vi "Main_v2.0.vi"() -> ()   [LabVIEW 2018]
doc: "This template is for the Queued Message Handler design pattern.\n\nThe Event Handling Loop generates messages based on user interface actions.\n\nThe Message Handling Loop processes messages generated by the Event Handling Loop, or by other messages. The messages are string values, so new messages can be added easily to the Message Cases case structure in the Message Handling Loop. Each message cluster can also provide an optional value for Message Data, which is a variant that can be converted to whatever message-specific data is required."
uses:
  Data_Type Def.ctl
  <vilib>/DAQmx/read.llb/DAQmx Read (Analog 1D DBL 1Chan NSamp).vi
  Global Variables.vi
  Enqueue Message (Single).vi
  <vilib>/measure/macond.llb/FIR Filter for 1 Chan.vi
  <vilib>/addons/Time Series Analysis/Statistical Analysis.llb/TSA Mean (Waveform).vi
  <vilib>/Utility/file.llb/Write Delimited Spreadsheet (DBL).vi
  <vilib>/DAQmx/create/channels.llb/DAQmx Create Channel (AI-Voltage-Basic).vi
  <vilib>/DAQmx/configure/timing.llb/DAQmx Timing (Sample Clock).vi
  <vilib>/DAQmx/configure/trigger.llb/DAQmx Start Trigger (Digital Edge).vi
  <vilib>/DAQmx/miscellaneous.llb/DAQmx Fill In Error Info.vi
  Message Queue.lvlib
  User Event - Stop.lvlib
  <resource>/objmgr/daqmx.rc
  <vilib>/measure/NI_MAPro.lvlib
  <vilib>/addons/_Advanced Signal Processing/NI_AdvSigProcTSA.lvlib
panel:
  out "Global Cos Corrected":T1(plugin-control)
  in  "Z dim (mm)":dbl=81.8
  out "Image array":dbl[][](array[numeric])
  in  "Experiment Name":string="v1_3x3_rep-1"
  out "Base File Name":string
  out "Points measured":i32
  in  "Trigger form CNC":tag="/DAQ2/PFI7"
  in  "Bleed (mm)":dbl=3.0
  in  "STOP":bool
  out "RAW":T1(plugin-control)
  in  "Max Input (V)":dbl=0.5
  in  "Min Input (V)":dbl
  in  "Step (mm)":dbl=0.2
  in  "X dim (mm)":dbl=30.0
  in  "Y dim (mm)":dbl=30.0
  in  "Voltage input from photodiode":tag="DAQ2/ai0"
  in  "Start":bool
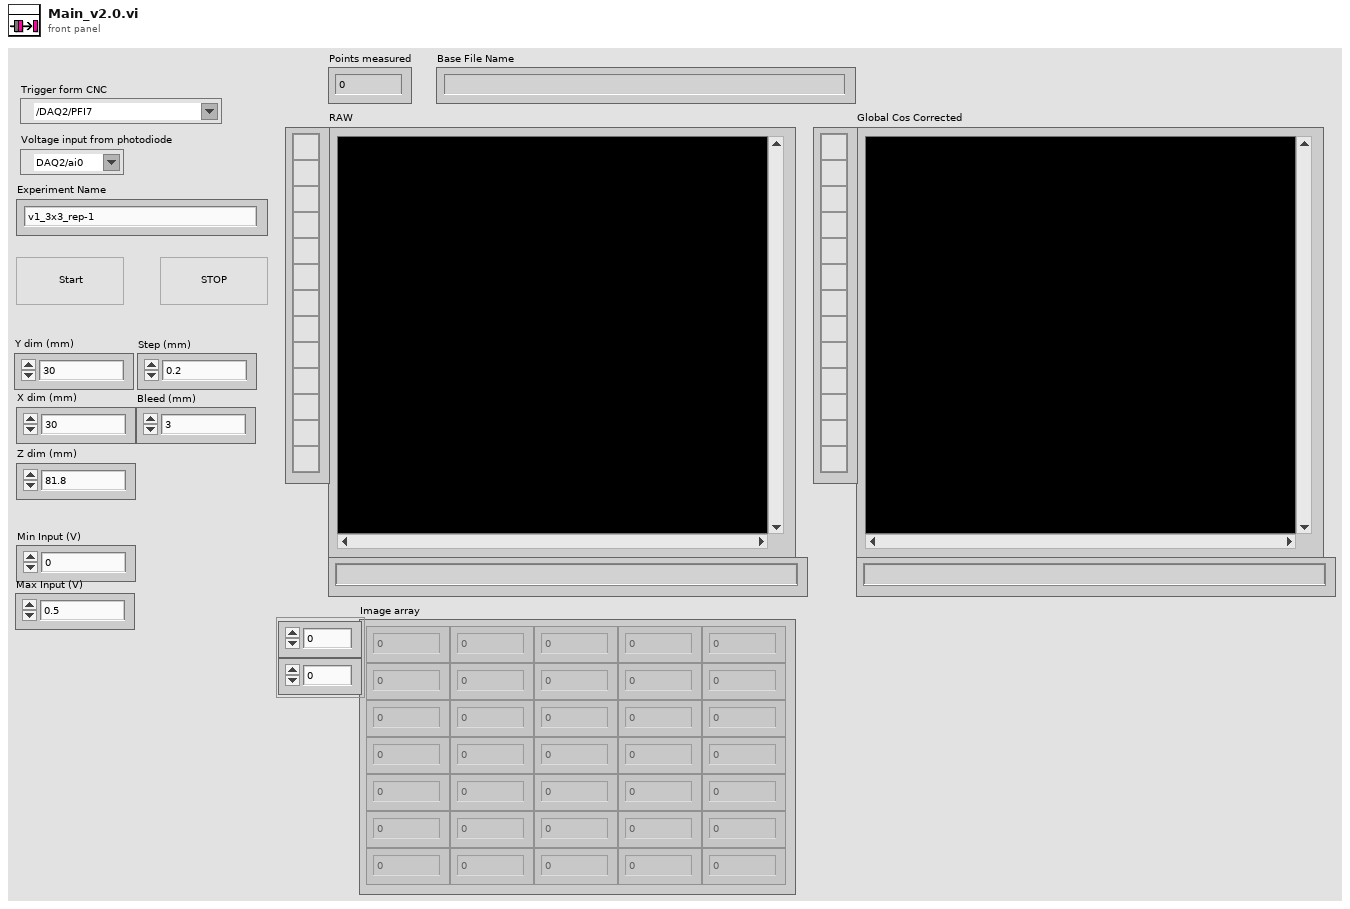
[diagram p1: front panel]
types:
  T1 = typedef "IMAQ Image.ctl" = refnum<image>
  T2 = typedef "Message Queue.lvlib/All Message Queues.ctl" = cluster{"Measurements":refnum<queue>, "Display":refnum<queue>}
  T3 = typedef "Data_Type Def.ctl" = cluster{"Data Array":dbl[], "Y iteration":i32, "X iteration":i32}
  T4 = cluster{"PB Gain":dbl, "SB Gain":dbl, "Scale":bool, "Window":enum16{"None", "Hanning", "Hamming", "Triangular", "Blackman", "Exact Blackman", "Blackman-Harris", "Kaiser-Bessel", "Flat Top"}}
  T5 = cluster{"Topology":enum16{"Off", "FIR by Specification", "Equi-ripple FIR", "Windowed FIR"}, "Type":enum16{"Lowpass", "Highpass", "Bandpass", "Bandstop"}, "#Taps":i32, "Lower PB":dbl, "Upper PB":dbl, "Lower SB":dbl, "Upper SB":dbl}
  T6 = typedef "Image Type" = u32
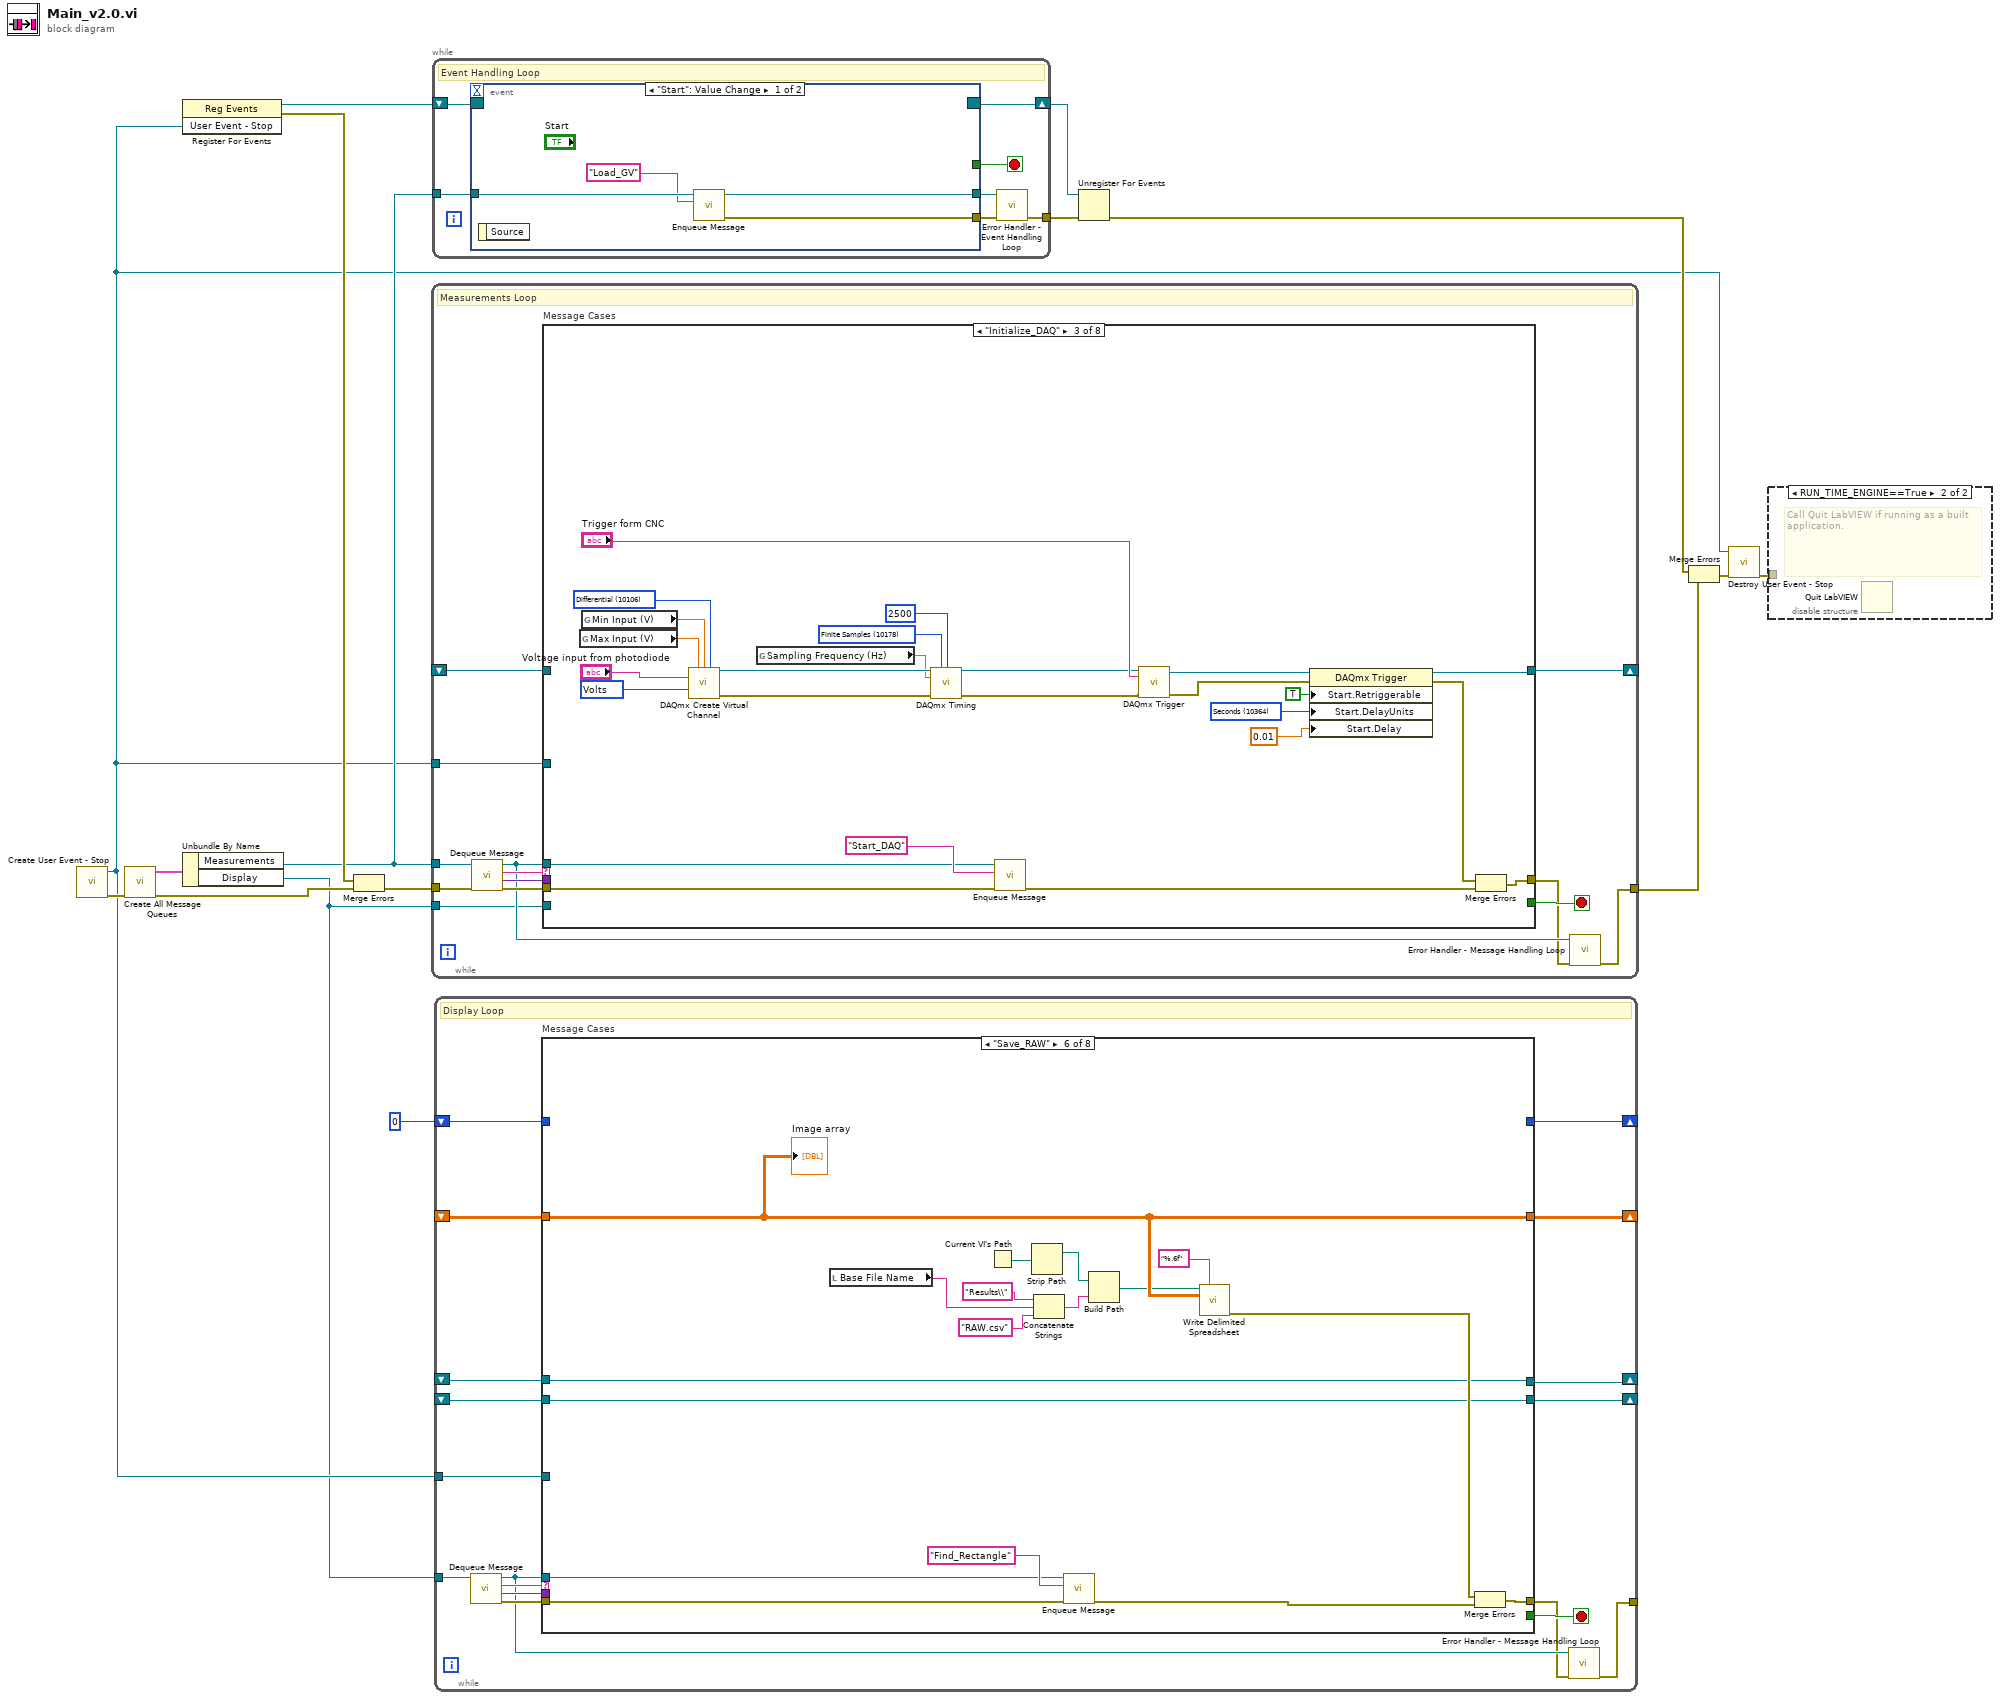
[diagram p0: block diagram]
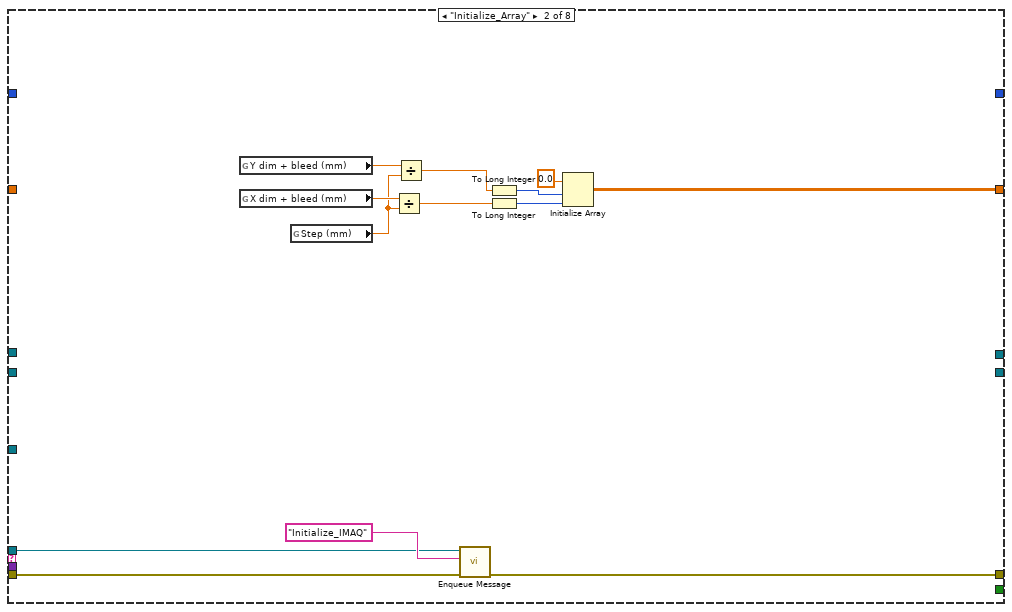
[diagram p3: hidden frame]
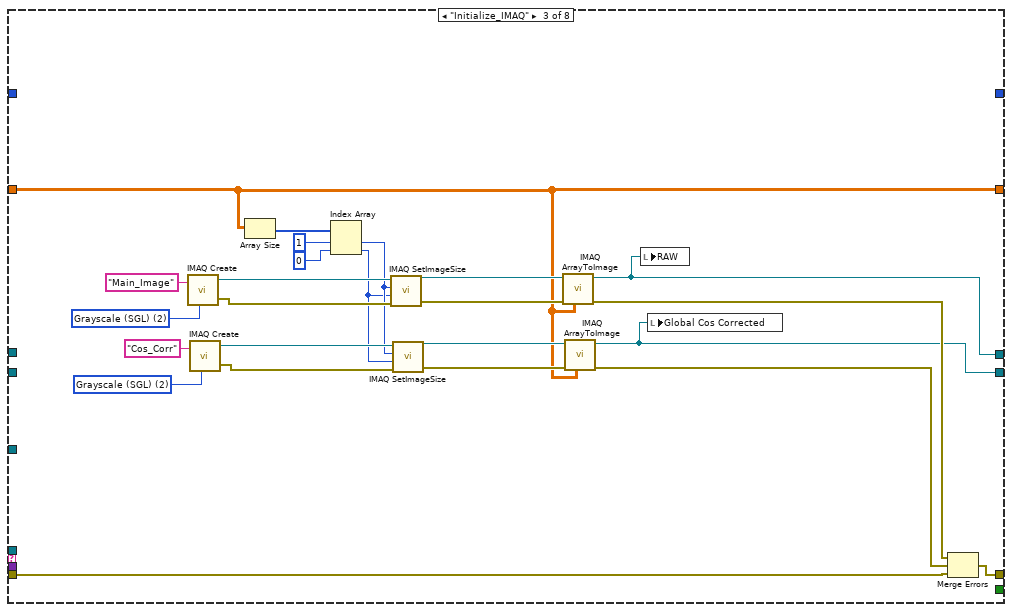
[diagram p4: hidden frame]
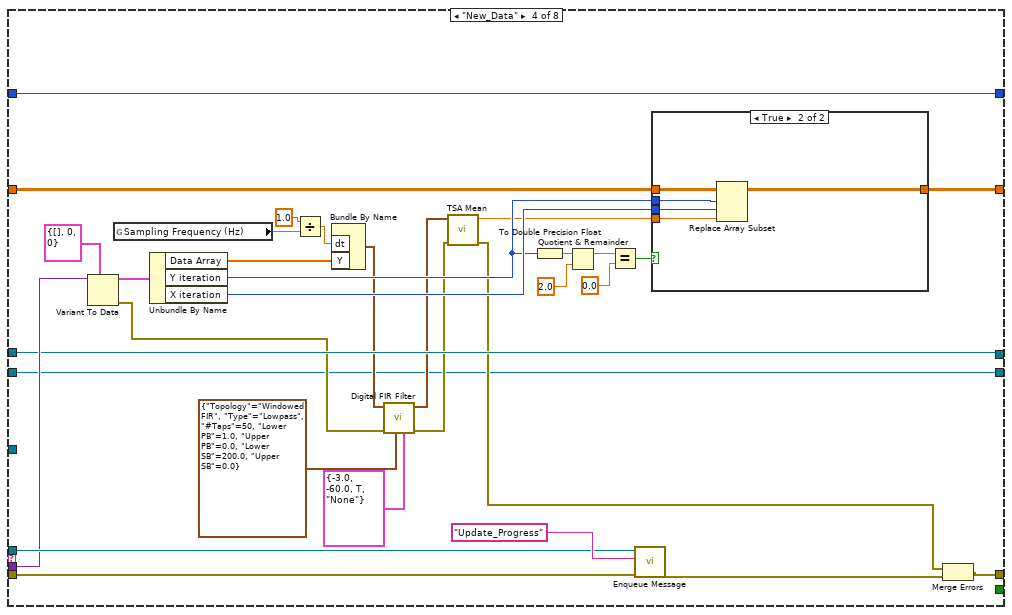
[diagram p5: hidden frame]
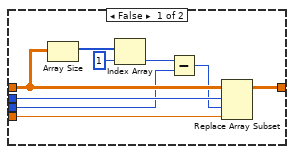
[diagram p6: hidden frame]
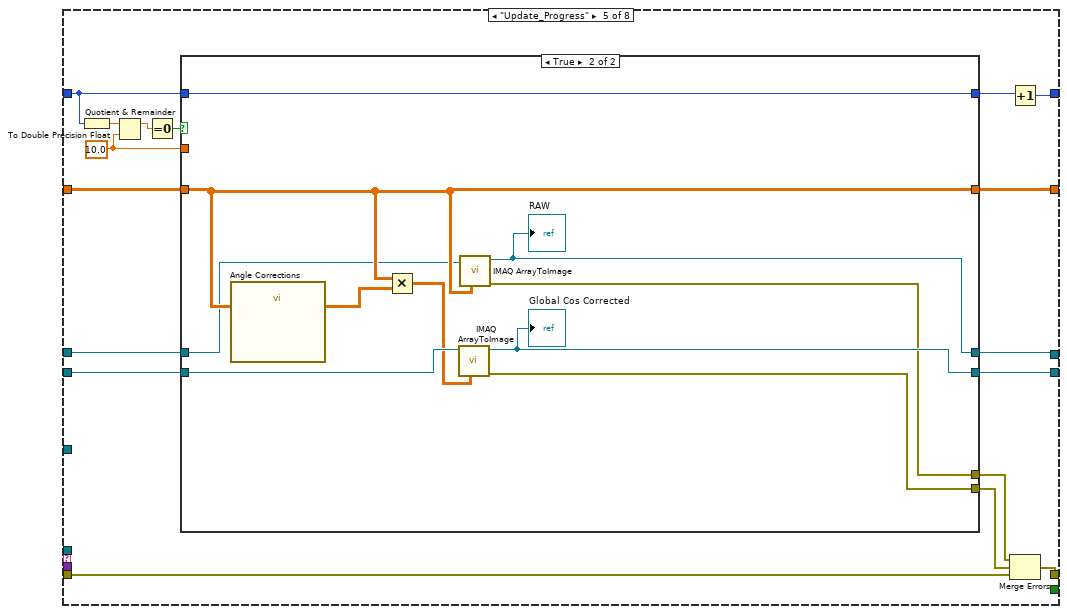
[diagram p7: hidden frame]
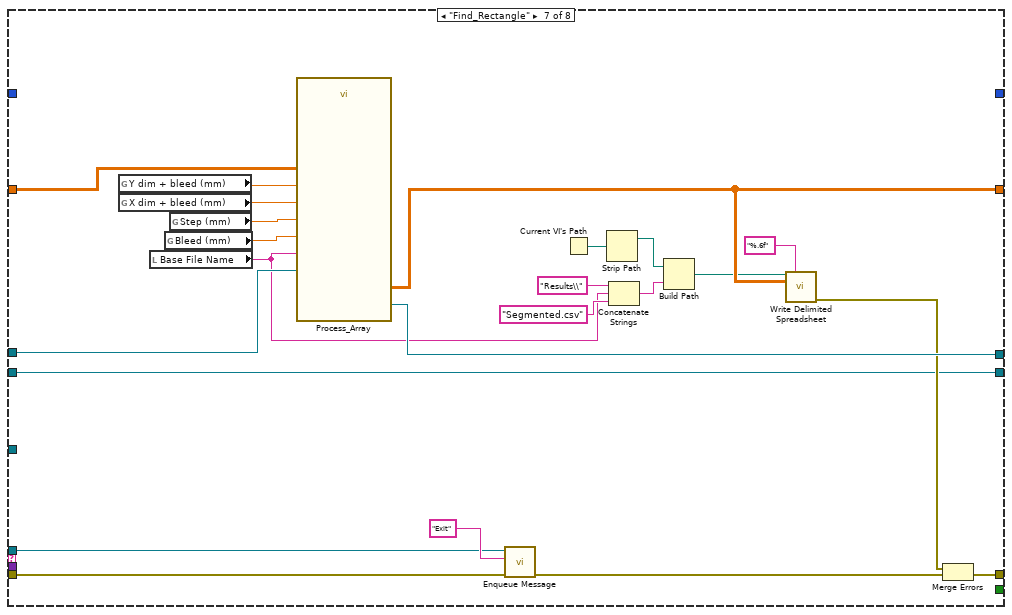
[diagram p9: hidden frame]
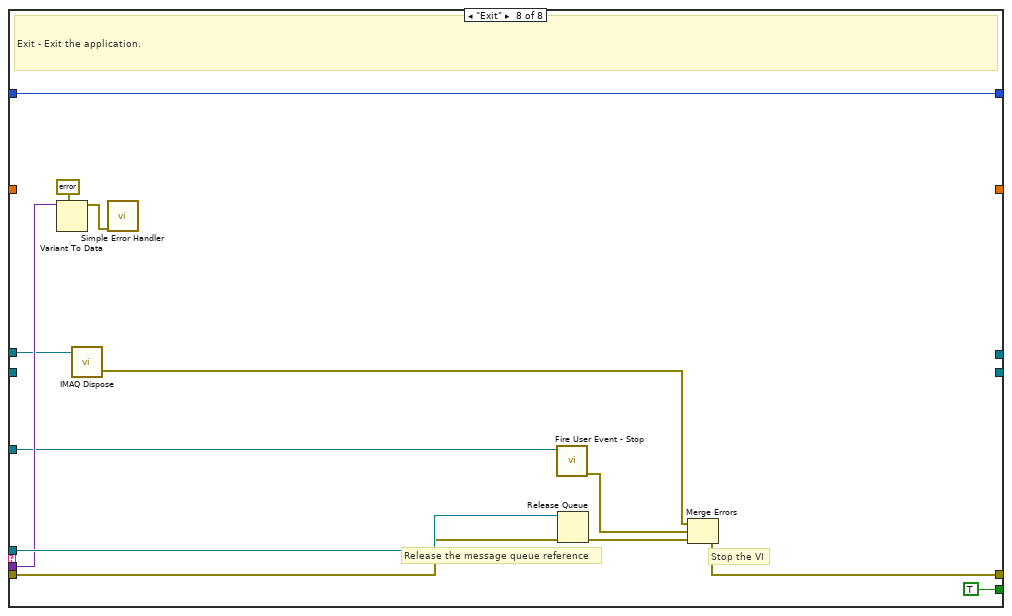
[diagram p10: hidden frame]
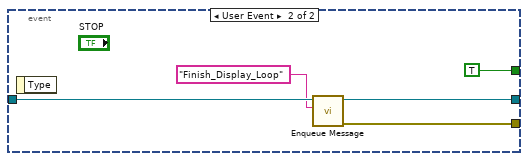
[diagram p12: hidden frame]
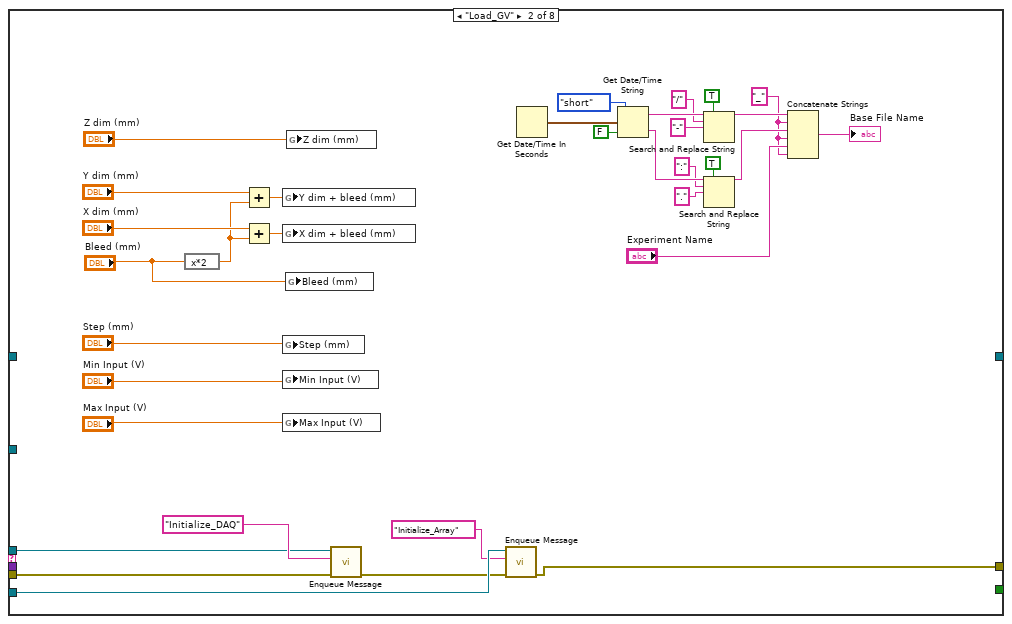
[diagram p14: hidden frame]
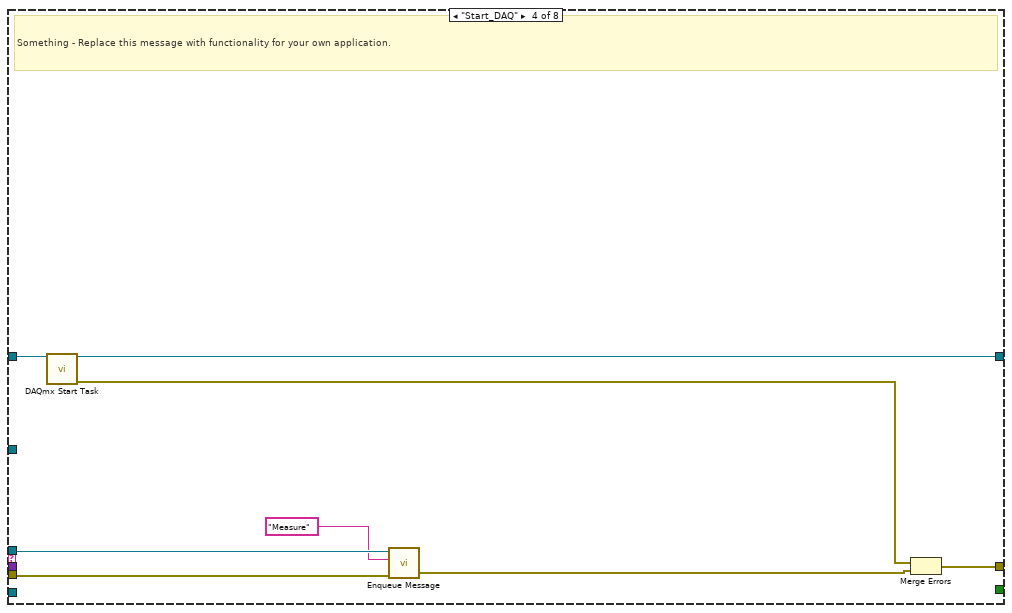
[diagram p15: hidden frame]
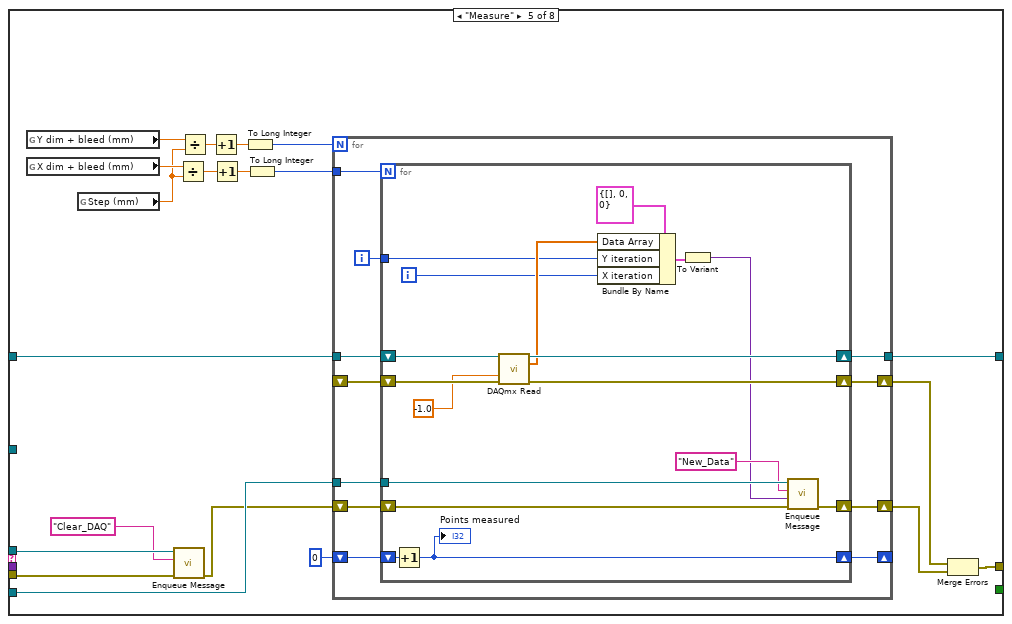
[diagram p16: hidden frame]
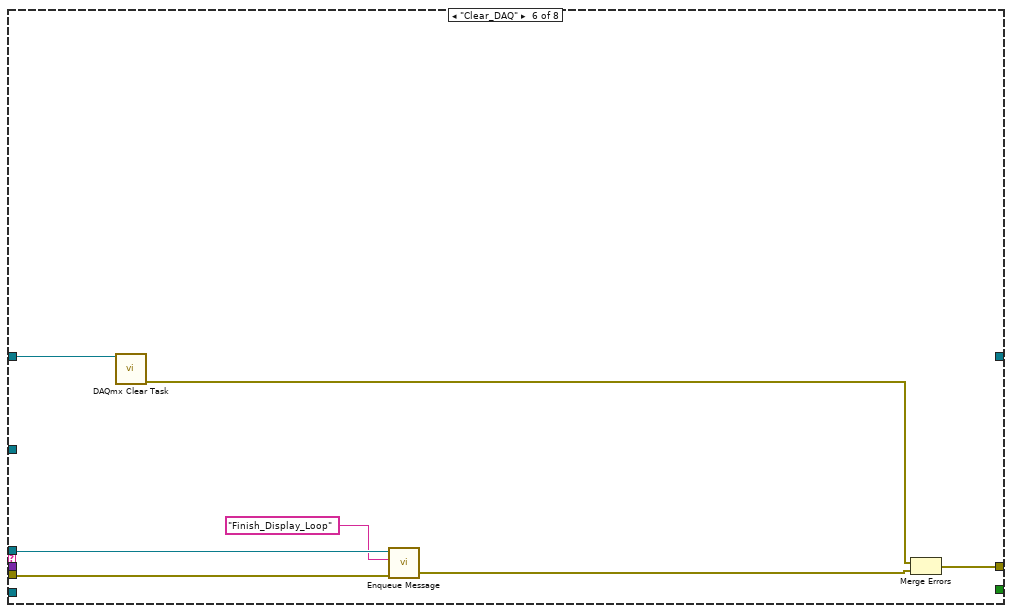
[diagram p17: hidden frame]
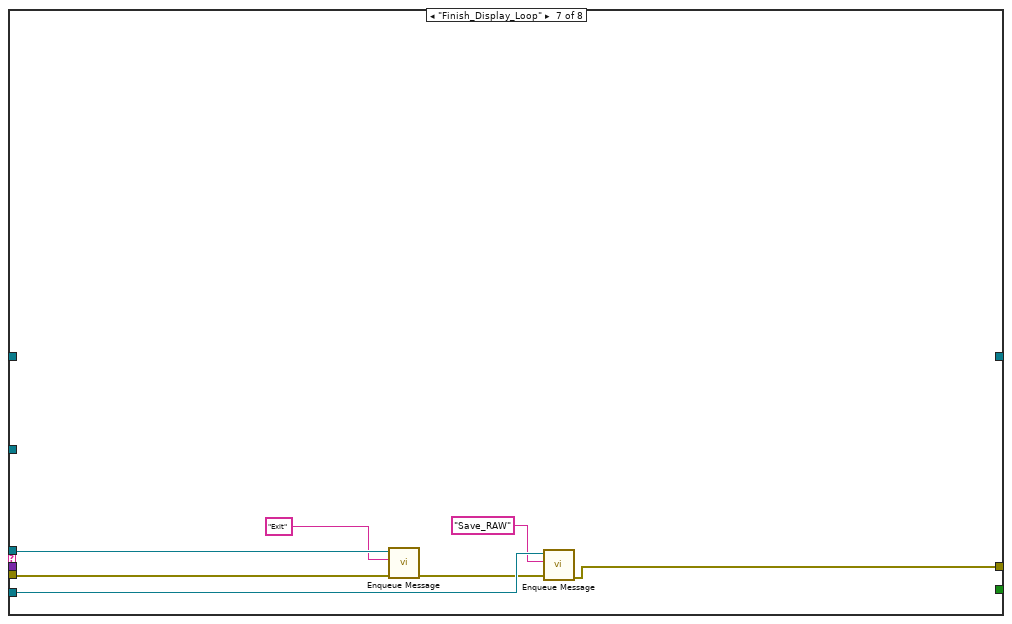
[diagram p18: hidden frame]
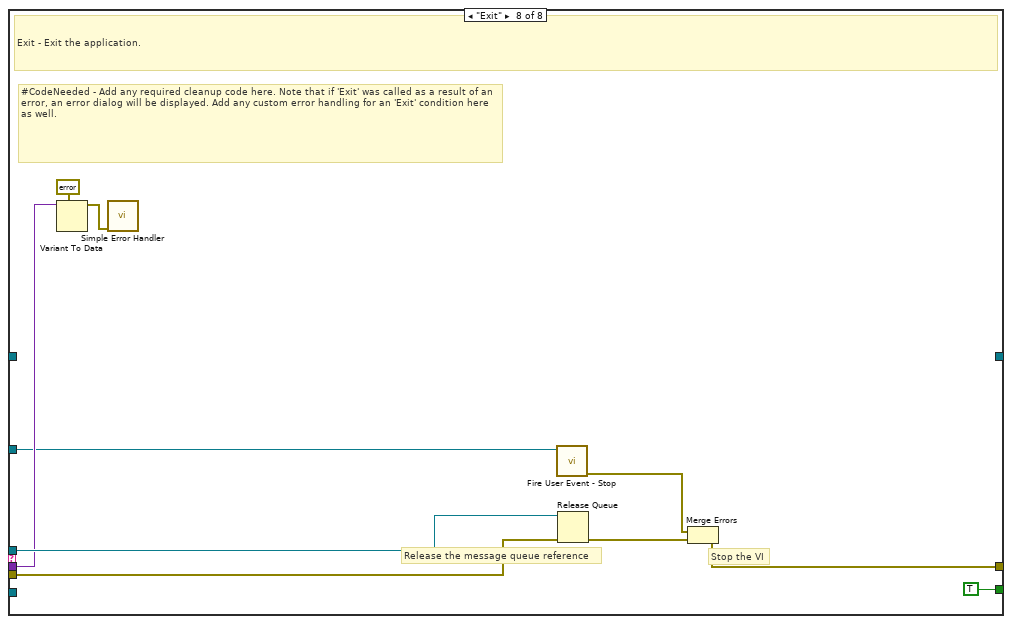
[diagram p19: hidden frame]
diagram:
  n1 = call "Create User Event - Stop.vi"() -> ("error out"=w13:errorcluster, "User Event - Stop"=w3:refnum<user-event>)  [unwired: 10 in]
  n2 = call "Create All Message Queues.vi"("error in (no error)"=w13) -> ("error out"=w16:errorcluster, "Message Queues out"=w15:T2)  [unwired: 9 in]
  n3 = register-events(w3) -> (reference out=w7:refnum<event-registration>, error out=w5:errorcluster)  [unwired: 2 in]
  n4 = Unbundle By Name(w15) -> ("Measurements"=w4:refnum<queue>, "Display"=w2:refnum<queue>)
  n5 = Merge Errors(w5, w16) -> (w6:errorcluster)
  n6 = while {
    tunnel: w4 -> [w24]
    tunnel: w6 -> [w28]
    tunnel: [w22] -> w14
    tunnel: w3 -> [w20]
    shift-right: [w19] -> _
    shift-left: _ -> [w17]
    tunnel: w2 -> [w18]
    stop <- w29 stop-if-true
    # "Measurements Loop"
    n7 = call "Dequeue Message.vi"("error in (no error)"=w28, "Message Queue"=w24) -> ("error out"=w27:errorcluster, "Message Data"=w25:variant, "Message"=w26:string, "dup Message Queue"=w23:refnum<queue>)  [unwired: 6 in]
    n8 = case "Message Cases" shown="\"Initialize_DAQ\"" w26 {
      tunnel: w23 -> [_ w62 w86 w93 w114 w148 w157 w168]
      tunnel: w27 -> [w30 w61 w88 w95 w115 w150 w158 w163]
      tunnel: [w30 w55 w78 w96 w116 w151 w152 w165] -> w21
      tunnel: [_ _ _ _ _ _ _ TRUE] -> w29
      tunnel: w25 -> [_ _ _ _ _ _ _ w160]
      tunnel: w20 -> [_ _ _ _ _ _ _ w159]
      tunnel: [_ _ w71 w90 w111 _ _ _] -> w19
      tunnel: w18 -> [_ w57 _ _ w100 _ w155 _]
      tunnel: w17 -> [_ _ _ w91 w112 w146 _ _]
      frame "Idle", Default {
      }
      frame "Load_GV" {
        w32 = "_" ("string")
        n9 = expression code="x*2"("Bleed (mm)") -> (w49:dbl)
        n10 = Add(x="Y dim (mm)", y=w49) -> (x+y=w53:dbl)
        n11 = Add(x="X dim (mm)", y=w49) -> (x+y=w52:dbl)
        n12 = global write "Global Variables.vi" "Y dim + bleed (mm)"(w53) -> ()
        n13 = global write "Global Variables.vi" "X dim + bleed (mm)"(w52) -> ()
        n14 = global write "Global Variables.vi" "Step (mm)"("Step (mm)") -> ()
        n15 = global write "Global Variables.vi" "Min Input (V)"("Min Input (V)") -> ()
        n16 = global write "Global Variables.vi" "Max Input (V)"("Max Input (V)") -> ()
        n17 = global write "Global Variables.vi" "Bleed (mm)"("Bleed (mm)") -> ()
        n18 = global write "Global Variables.vi" "Z dim (mm)"("Z dim (mm)") -> ()
        n19 = call-poly "Enqueue Message.vi"("error in (no error)"=w61, "Message"="Initialize_DAQ", "Message Queue"=w62) -> ("error out"=w56:errorcluster)  [unwired: 7 in, 1 out]
        n20 = call-poly "Enqueue Message.vi"("error in (no error)"=w56, "Message"="Initialize_Array", "Message Queue"=w57) -> ("error out"=w55:errorcluster)  [unwired: 7 in, 1 out]
        n21 = Get Date/Time In Seconds() -> (seconds since 1Jan1904=w47:timestamp)
        n22 = Get Date/Time String(date format (0)=enum16{"short", "long", "abbreviated"}."short", seconds (now)=w47, want seconds? (F)=FALSE) -> (date string=w44:string, time string=w37:string)
        n23 = Search and Replace String(replace all?=TRUE ("replace all? (F)"), input string=w44, search string="/", replace string="-" ("replace string (\"\")")) -> (result string=w40:string)  [unwired: 4 in, 3 out]
        n24 = Search and Replace String(replace all?=TRUE ("replace all? (F)"), input string=w37, search string=":", replace string="." ("replace string (\"\")")) -> (result string=w36:string)  [unwired: 4 in, 3 out]
        n25 = Concatenate Strings(w40, w32, w36, w32, "Experiment Name", w32) -> (→"Base File Name":string)
      }
      frame "Initialize_DAQ" {
        w67 = 10364 items=["Sample Clock Periods"=10286, "Seconds"=10364, "Ticks"=10304] ("Start.DelayUnits")
        w82 = 10178 items=["Finite Samples"=10178, "Continuous Samples"=10123, "Hardware Timed Single Point"=12522] ("sample mode")
        w83 = 10348 items=["Volts"=10348, "From Custom Scale"=10065] ("units")
        w85 = 10106 items=["Default"=-1, "RSE"=10083, "NRSE"=10078, "Differential"=10106, "Pseudodifferential"=12529] ("input terminal configuration")
        n26 = global read "Global Variables.vi" "Max Input (V)"() -> (w75:dbl)
        n27 = global read "Global Variables.vi" "Min Input (V)"() -> (w76:dbl)
        n28 = call-poly <vilib>:"DAQmx Create Virtual Channel.vi"("maximum value"=w75, "minimum value"=w76, "input terminal configuration"=w85, "physical channels"="Voltage input from photodiode", "units"=w83) -> ("task out"=w81:refnum<k21>, "error out"=w80:errorcluster)  [unwired: 9 in]
        n29 = global read "Global Variables.vi" "Sampling Frequency (Hz)"() -> (w64:dbl)
        n30 = call-poly <vilib>:"DAQmx Timing.vi"("task/channels in"=w81, "sample mode"=w82, "samples per channel"=2500, "rate"=w64, "error in"=w80) -> ("task out"=w65:refnum<k21>, "error out"=w74:errorcluster)  [unwired: 9 in]
        n31 = call-poly "Enqueue Message.vi"("error in (no error)"=w88, "Message"="Start_DAQ", "Message Queue"=w86) -> ("error out"=w77:errorcluster)  [unwired: 7 in, 1 out]
        n32 = call-poly <vilib>:"DAQmx Trigger.vi"("task/channels in"=w65, "source"="Trigger form CNC", "error in"=w74) -> ("task out"=w69:refnum<k21>, "error out"=w72:errorcluster)  [unwired: 11 in]
        n33 = property class="DAQmx Trigger"(reference=w69, error in=w72, "Start.Retriggerable"=TRUE, "Start.DelayUnits"=w67, "Start.Delay"=0.01) -> (reference out=w71:refnum<k21>, error out=w70:errorcluster)
        n34 = Merge Errors(w70, w77) -> (w78:errorcluster)
      }
      frame "Start_DAQ" {
        # "Something - Replace this message with functionality for your own application."
        n35 = call <vilib>:"DAQmx Start Task.vi"("task/channels in"=w91) -> ("task out"=w90:refnum<k21>, "error out"=w89:errorcluster)  [unwired: 13 in]
        n36 = call-poly "Enqueue Message.vi"("error in (no error)"=w95, "Message"="Measure", "Message Queue"=w93) -> ("error out"=w94:errorcluster)  [unwired: 7 in, 1 out]
        n37 = Merge Errors(w89, w94) -> (w96:errorcluster)
      }
      frame "Measure" {
        n38 = global read "Global Variables.vi" "Y dim + bleed (mm)"() -> (w106:dbl)
        n39 = global read "Global Variables.vi" "X dim + bleed (mm)"() -> (w105:dbl)
        n40 = global read "Global Variables.vi" "Step (mm)"() -> (w104:dbl)
        n41 = call-poly "Enqueue Message.vi"("error in (no error)"=w115, "Message"="Clear_DAQ", "Message Queue"=w114) -> ("error out"=w99:errorcluster)  [unwired: 7 in, 1 out]
        n42 = Divide(x=w105, y=w104) -> (x/y=w109:dbl)
        n43 = Divide(x=w106, y=w104) -> (x/y=w110:dbl)
        n44 = Increment(x=w110) -> (x+1=w108:dbl)
        n45 = Increment(x=w109) -> (x+1=w107:dbl)
        n46 = To Long Integer(number=w108) -> (32bit integer=w102:i32)
        n47 = To Long Integer(number=w107) -> (32bit integer=w101:i32)
        n48 = for {
          N: w102 -> [_]
          tunnel: w112 -> [w127]
          tunnel: [w126] -> w111
          shift-right: [w125] -> w103
          shift-left: _ -> [w124]
          tunnel: w101 -> [w123]
          tunnel: w100 -> [w122]
          shift-right: [w120] -> w98
          shift-left: w99 -> [w121]
          shift-right: [w117] -> _
          shift-left: 0 -> [w118]
          i -> [w119]
          n49 = for {
            N: w123 -> [_]
            shift-right: [w143] -> w126
            shift-left: w127 -> [w144]
            shift-right: [w142] -> w125
            shift-left: w124 -> [w141]
            tunnel: w122 -> [w140]
            shift-right: [w137] -> w120
            shift-left: w121 -> [w138]
            tunnel: w119 -> [w133]
            shift-right: [w128] -> w117
            shift-left: w118 -> [w129]
            i -> [w132]
            n50 = Increment(x=w129) -> (x+1=w128:i32)
            "Points measured" <- w128
            n51 = call-poly <vilib>:"DAQmx Read.vi"("task/channels in"=w144, "timeout"=-1.0, "error in"=w141) -> ("task out"=w143:refnum<k21>, "data"=w134:dbl[], "error out"=w142:errorcluster)  [unwired: 10 in]
            n52 = Bundle By Name(cluster=T3 {"Data Array"=[], "Y iteration"=0, "X iteration"=0}, "Data Array"=w134, "Y iteration"=w133, "X iteration"=w132) -> (w131:T3)
            n53 = To Variant(anything=w131) -> (Variant=w136:variant)
            n54 = call-poly "Enqueue Message.vi"("error in (no error)"=w138, "Message Data"=w136, "Message"="New_Data", "Message Queue"=w140) -> ("error out"=w137:errorcluster)  [unwired: 6 in, 1 out]
          }
        }
        n55 = Merge Errors(w103, w98) -> (w116:errorcluster)
      }
      frame "Clear_DAQ" {
        n56 = call <vilib>:"DAQmx Clear Task.vi"("task in"=w146) -> ("error out"=w145:errorcluster)  [unwired: 14 in]
        n57 = call-poly "Enqueue Message.vi"("error in (no error)"=w150, "Message"="Finish_Display_Loop", "Message Queue"=w148) -> ("error out"=w149:errorcluster)  [unwired: 7 in, 1 out]
        n58 = Merge Errors(w145, w149) -> (w151:errorcluster)
      }
      frame "Finish_Display_Loop" {
        n59 = call-poly "Enqueue Message.vi"("error in (no error)"=w158, "Message"="Exit", "Message Queue"=w157) -> ("error out"=w154:errorcluster)  [unwired: 7 in, 1 out]
        n60 = call-poly "Enqueue Message.vi"("error in (no error)"=w154, "Message"="Save_RAW", "Message Queue"=w155) -> ("error out"=w152:errorcluster)  [unwired: 7 in, 1 out]
      }
      frame "Exit" {
        # "Stop the VI"
        # "Release the message queue reference"
        # "#CodeNeeded - Add any required cleanup code here. Note that if 'Exit' was called as a result of an error, an error dialog will be displayed. Add any custom error handling for an 'Exit' condition here as well."
        # "Exit - Exit the application."
        n61 = Variant To Data(type=errorcluster {"status"=FALSE, "code"=0, "source"=""} ("error constant"), Variant=w160) -> (data=w161:errorcluster)  [unwired: 1 in, 1 out]
        n62 = call <vilib>:"Simple Error Handler.vi"("error in (no error)"=w161) -> ()  [unwired: 4 in, 5 out]
        n63 = call "Fire User Event - Stop.vi"("User Event - Stop"=w159) -> ("error out"=w164:errorcluster)  [unwired: 10 in]
        n64 = Release Queue(queue=w168, error in (no error)=w163) -> (error out=w166:errorcluster)  [unwired: 1 in, 2 out]
        n65 = Merge Errors(w164, w166) -> (w165:errorcluster)
      }
    }
    n66 = call "Error Handler - Message Handling Loop.vi"("error in (no error)"=w21, "Message Queue"=w23) -> ("dup error in"=w22:errorcluster)  [unwired: 8 in, 1 out]
  }
  n67 = while {
    tunnel: w4 -> [w175]
    shift-right: [w173] -> w10
    shift-left: w7 -> [w174]
    tunnel: [w169] -> w8
    stop <- w171 stop-if-true
    # "Event Handling Loop"
    n68 = event shown="[0] \"Start\": Value Change" {
      selector: w174 -> [_ _]
      dyn-events: [_ _] -> w173
      timeout: _ -> [_ _]
      tunnel: [_ TRUE ("Discard?")] -> w171
      tunnel: w175 -> [w179 w183]
      tunnel: [w176 w181] -> w172
      tunnel: [w178 w182] -> w170
      event "Start": Value Change {
        n69 = event-data() -> ()  [unwired: 1 in, 1 out]
        n70 = call-poly "Enqueue Message.vi"("Message"="Load_GV", "Message Queue"=w179) -> ("error out"=w176:errorcluster, "dup Message Queue"=w178:refnum<queue>)  [unwired: 8 in]
      }
      event User Event {
        n71 = event-data() -> ()  [unwired: 1 in, 1 out]
        n72 = call-poly "Enqueue Message.vi"("Message"="Finish_Display_Loop" ("VI Stopped"), "Message Queue"=w183) -> ("error out"=w181:errorcluster, "dup Message Queue"=w182:refnum<queue>)  [unwired: 8 in]
      }
    }
    n73 = call "Error Handler - Event Handling Loop.vi"("error in (no error)"=w172, "Message Queue"=w170) -> ("dup error in"=w169:errorcluster)  [unwired: 8 in, 1 out]
  }
  n74 = while {
    tunnel: w2 -> [w197]
    tunnel: [w195] -> _
    tunnel: w3 -> [w193]
    shift-right: [w192] -> _
    shift-left: _ -> [w187]
    shift-right: [w190] -> _
    shift-left: 0 -> [w191]
    shift-right: [w189] -> _
    shift-left: _ -> [w188]
    shift-right: [w186] -> _
    shift-left: _ -> [w185]
    stop <- w201 stop-if-true
    # "Display Loop"
    n75 = call "Dequeue Message.vi"("Message Queue"=w197) -> ("error out"=w200:errorcluster, "Message Data"=w198:variant, "Message"=w199:string, "dup Message Queue"=w196:refnum<queue>)  [unwired: 7 in]
    n76 = case "Message Cases" shown="\"Save_RAW\"" w199 {
      tunnel: w196 -> [_ w207 _ w269 _ w327 w342 w369]
      tunnel: w200 -> [w202 w206 w216 w271 w286 w328 w341 w364]
      tunnel: [w202 w205 w235 w248 w298 w333 w345 w366] -> w194
      tunnel: [_ _ _ _ _ _ _ TRUE] -> w201
      tunnel: w198 -> [_ _ _ w268 _ _ _ w361]
      tunnel: w193 -> [_ _ _ _ _ _ _ w360]
      tunnel: [_ w209 w217 w259 w301 w325 w346 _] -> w192
      tunnel: w187 -> [_ _ w217 w258 w302 w325 w335 _]
      tunnel: w191 -> [_ _ _ w265 w294 _ _ w359]
      tunnel: [_ _ _ w265 w296 _ _ w359] -> w190
      tunnel: [_ _ w229 w255 w299 w326 w351 _] -> w189
      tunnel: w188 -> [_ _ _ w255 w300 w326 w352 w358]
      tunnel: [_ _ w218 w240 w289 w317 w334 _] -> w186
      tunnel: w185 -> [_ _ _ w240 w290 w317 w334 _]
      frame "Idle", Default {
      }
      frame "Initialize_Array" {
        n77 = global read "Global Variables.vi" "Y dim + bleed (mm)"() -> (w214:dbl)
        n78 = global read "Global Variables.vi" "X dim + bleed (mm)"() -> (w213:dbl)
        n79 = global read "Global Variables.vi" "Step (mm)"() -> (w212:dbl)
        n80 = Divide(x=w213, y=w212) -> (x/y=w203:dbl)
        n81 = Divide(x=w214, y=w212) -> (x/y=w204:dbl)
        n82 = call-poly "Enqueue Message.vi"("error in (no error)"=w206, "Message"="Initialize_IMAQ", "Message Queue"=w207) -> ("error out"=w205:errorcluster)  [unwired: 7 in, 1 out]
        n83 = To Long Integer(number=w204) -> (32bit integer=w210:i32)
        n84 = To Long Integer(number=w203) -> (32bit integer=w211:i32)
        n85 = Initialize Array(0.0, w210, w211) -> (w209:dbl[][])
      }
      frame "Initialize_IMAQ" {
        w227 = T6 2 items=["Grayscale (U8)", "Grayscale (I16)", "Grayscale (SGL)", "Complex (CSG)", "RGB (U32)", "HSL (U32)", "RGB (U64)", "Grayscale (U16)"] ("Image Type")
        w238 = T6 2 items=["Grayscale (U8)", "Grayscale (I16)", "Grayscale (SGL)", "Complex (CSG)", "RGB (U32)", "HSL (U32)", "RGB (U64)", "Grayscale (U16)"] ("Image Type")
        n86 = call "IMAQ Create"("Image Name"="Main_Image", "Image Type"=w238) -> ("New Image"=w237:T1, "error out"=w236:errorcluster)  [unwired: 3 in]
        n87 = call "IMAQ Create"("Image Name"="Cos_Corr", "Image Type"=w227) -> ("New Image"=w226:T1, "error out"=w225:errorcluster)  [unwired: 3 in]
        n88 = Array Size(array=w217) -> (size(s)=w234:i32[])
        n89 = Index Array(array=w234, index #1=1 ("index"), index #2=0 ("index")) -> (element #1=w222:i32, element #2=w221:i32)
        n90 = call "IMAQ SetImageSize"("error in (no error)"=w236, "Y Resolution"=w221, "X Resolution"=w222, "Image"=w237) -> ("error out"=w231:errorcluster, "Image Out"=w230:T1)  [unwired: 1 in]
        n91 = call "IMAQ SetImageSize"("error in (no error)"=w225, "Y Resolution"=w221, "X Resolution"=w222, "Image"=w226) -> ("error out"=w224:errorcluster, "Image Out"=w223:T1)  [unwired: 1 in]
        n92 = call "IMAQ ArrayToImage"("Image Pixels (Float)"=w217, "error in (no error)"=w231, "Image"=w230) -> ("error out"=w220:errorcluster, "Image Out"=w229:T1)  [unwired: 7 in]
        n93 = call "IMAQ ArrayToImage"("Image Pixels (Float)"=w217, "error in (no error)"=w224, "Image"=w223) -> ("error out"=w219:errorcluster, "Image Out"=w218:T1)  [unwired: 7 in]
        n94 = local write "RAW"(w229) -> ()
        n95 = local write "Global Cos Corrected"(w218) -> ()
        n96 = Merge Errors(w220, w219, w216) -> (w235:errorcluster)
      }
      frame "New_Data" {
        n97 = Variant To Data(type=T3 {"Data Array"=[], "Y iteration"=0, "X iteration"=0}, Variant=w268) -> (data=w266:T3, error out=w249:errorcluster)  [unwired: 1 in]
        n98 = global read "Global Variables.vi" "Sampling Frequency (Hz)"() -> (w242:dbl)
        n99 = Unbundle By Name(w266) -> ("Data Array"=w245:dbl[], "Y iteration"=w256:i32, "X iteration"=w257:i32)
        n100 = Divide(x=1.0, y=w242) -> (x/y=w243:dbl)
        n101 = Bundle By Name("dt"=w243, "Y"=w245) -> (w244:waveform(dbl))  [unwired: 1 in]
        n102 = call-poly <vilib>:"Digital FIR Filter.vi"("optional FIR filter specifications"=T4 {"PB Gain"=-3.0, "SB Gain"=-60.0, "Scale"=TRUE, "Window"=enum."None"}, "FIR filter specifications"=T5 {"Topology"=enum."Windowed FIR", "Type"=enum."Lowpass", "#Taps"=50, "Lower PB"=1.0, "Upper PB"=0.0, "Lower SB"=200.0, "Upper SB"=0.0}, "error in (no error)"=w249, "signal in"=w244) -> ("error out"=w250:errorcluster, "signal out"=w252:waveform(dbl))  [unwired: 5 in, 1 out]
        n103 = call-poly <vilib>:"TSA Mean.vi"("error in (no error)"=w250, "Xt"=w252) -> ("error out"=w246:errorcluster, "mean"=w251:dbl)  [unwired: 8 in]
        n104 = To Double Precision Float(number=w256) -> (double precision float=w262:dbl)
        n105 = Quotient & Remainder(x=w262, y=2.0) -> (x-y*floor(x/y)=w263:dbl)  [unwired: 1 out]
        n106 = Equal?(x=w263, y=0.0) -> (x = y?=w264:bool)
        n107 = call-poly "Enqueue Message.vi"("error in (no error)"=w271, "Message"="Update_Progress", "Message Queue"=w269) -> ("error out"=w247:errorcluster)  [unwired: 7 in, 1 out]
        n108 = case shown="True" w264 {
          tunnel: [w280 w285] -> w259
          tunnel: w258 -> [w277 w284]
          tunnel: w251 -> [w279 w283]
          tunnel: w257 -> [w274 w282]
          tunnel: w256 -> [w278 w281]
          frame False {
            n109 = Array Size(array=w277) -> (size(s)=w276:i32[])
            n110 = Index Array(array=w276, index=1) -> (element=w275:i32)
            n111 = Subtract(x=w275, y=w274) -> (x-y=w273:i32)
            n112 = Replace Array Subset(array=w277, new element=w279, index (row)=w278, index (col)=w273) -> (w280:dbl[][])
          }
          frame True {
            n113 = Replace Array Subset(array=w284, new element=w283, index (row)=w281, index (col)=w282) -> (w285:dbl[][])
          }
        }
        n114 = Merge Errors(w246, w247) -> (w248:errorcluster)
      }
      frame "Update_Progress" {
        w291 = 10.0 ("y")
        n115 = To Double Precision Float(number=w294) -> (double precision float=w295:dbl)
        n116 = Quotient & Remainder(x=w295, y=w291) -> (x-y*floor(x/y)=w293:dbl)  [unwired: 1 out]
        n117 = Equal To 0?(x=w293) -> (x = 0?=w292:bool)
        n118 = case shown="True" w292 {
          tunnel: w294 -> [w304 w316]
          tunnel: [w304 w316] -> w297
          tunnel: w302 -> [w306 w312]
          tunnel: [w306 w312] -> w301
          tunnel: w300 -> [w305 w309]
          tunnel: [w305 w315] -> w299
          tunnel: w291 -> [_ _]
          tunnel: w290 -> [w303 w308]
          tunnel: [w303 w314] -> w289
          tunnel: [_ w311] -> w288
          tunnel: [_ w310] -> w287
          frame False {
          }
          frame True {
            n119 = call "Angle Corrections.vi"("Image array"=w312) -> ("Image array_Cos_Correction"=w313:dbl[][])  [unwired: 10 in]
            n120 = Multiply(x=w312, y=w313) -> (x*y=w307:dbl[][])
            n121 = call "IMAQ ArrayToImage"("Image Pixels (Float)"=w307, "Image"=w308) -> ("error out"=w310:errorcluster, "Image Out"=w314:T1)  [unwired: 8 in]
            "Global Cos Corrected" <- w314
            n122 = call "IMAQ ArrayToImage"("Image Pixels (Float)"=w312, "Image"=w309) -> ("error out"=w311:errorcluster, "Image Out"=w315:T1)  [unwired: 8 in]
            "RAW" <- w315
          }
        }
        n123 = Increment(x=w297) -> (x+1=w296:i32)
        n124 = Merge Errors(w288, w287, w286) -> (w298:errorcluster)
      }
      frame "Save_RAW" {
        n125 = local read "Base File Name"() -> (w320:string)
        n126 = Current VI's Path() -> (path=w318:path)
        n127 = Strip Path(path=w318) -> (stripped path=w322:path)  [unwired: 1 out]
        n128 = Concatenate Strings("Results\\" ("name or relative path"), w320, "RAW.csv" ("string")) -> (w321:string)
        n129 = call-poly "Enqueue Message.vi"("error in (no error)"=w328, "Message"="Find_Rectangle", "Message Queue"=w327) -> ("error out"=w329:errorcluster)  [unwired: 7 in, 1 out]
        n130 = Build Path(base path=w322, name or relative path=w321) -> (appended path=w319:path)
        n131 = call-poly <vilib>:"Write Delimited Spreadsheet.vi"("file path (dialog if empty)"=w319, "format (%.3f)"="%.6f", "2D data"=w325) -> ("error out"=w332:errorcluster)  [unwired: 11 in, 1 out]
        n132 = Merge Errors(w332, w329) -> (w333:errorcluster)
        "Image array" <- w325
      }
      frame "Find_Rectangle" {
        n133 = global read "Global Variables.vi" "Y dim + bleed (mm)"() -> (w356:dbl)
        n134 = global read "Global Variables.vi" "X dim + bleed (mm)"() -> (w355:dbl)
        n135 = local read "Base File Name"() -> (w347:string)
        n136 = global read "Global Variables.vi" "Bleed (mm)"() -> (w353:dbl)
        n137 = global read "Global Variables.vi" "Step (mm)"() -> (w354:dbl)
        n138 = call "Process_Array.vi"("Image array"=w335, "Base_name"=w347, "Image In"=w352, "Bleed (mm)"=w353, "Step (mm) 2"=w354, "X dim + bleed (mm)"=w355, "Y dim + bleed (mm)"=w356) -> ("Image array"=w346:dbl[][], "Image Out"=w351:T1)  [unwired: 3 in]
        n139 = call-poly "Enqueue Message.vi"("error in (no error)"=w341, "Message"="Exit", "Message Queue"=w342) -> ("error out"=w340:errorcluster)  [unwired: 7 in, 1 out]
        n140 = Current VI's Path() -> (path=w336:path)
        n141 = Strip Path(path=w336) -> (stripped path=w338:path)  [unwired: 1 out]
        n142 = Concatenate Strings("Results\\" ("name or relative path"), w347, "Segmented.csv" ("string")) -> (w337:string)
        n143 = Build Path(base path=w338, name or relative path=w337) -> (appended path=w339:path)
        n144 = call-poly <vilib>:"Write Delimited Spreadsheet.vi"("file path (dialog if empty)"=w339, "format (%.3f)"="%.6f", "2D data"=w346) -> ("error out"=w344:errorcluster)  [unwired: 11 in, 1 out]
        n145 = Merge Errors(w344, w340) -> (w345:errorcluster)
      }
      frame "Exit" {
        # "Stop the VI"
        # "Release the message queue reference"
        # "Exit - Exit the application."
        n146 = Variant To Data(type=errorcluster {"status"=FALSE, "code"=0, "source"=""} ("error constant"), Variant=w361) -> (data=w362:errorcluster)  [unwired: 1 in, 1 out]
        n147 = call "IMAQ Dispose"("Image"=w358) -> ("error out"=w357:errorcluster)  [unwired: 5 in]
        n148 = call <vilib>:"Simple Error Handler.vi"("error in (no error)"=w362) -> ()  [unwired: 4 in, 5 out]
        n149 = call "Fire User Event - Stop.vi"("User Event - Stop"=w360) -> ("error out"=w365:errorcluster)  [unwired: 10 in]
        n150 = Release Queue(queue=w369, error in (no error)=w364) -> (error out=w367:errorcluster)  [unwired: 1 in, 2 out]
        n151 = Merge Errors(w357, w365, w367) -> (w366:errorcluster)
      }
    }
    n152 = call "Error Handler - Message Handling Loop.vi"("error in (no error)"=w194, "Message Queue"=w196) -> ("dup error in"=w195:errorcluster)  [unwired: 8 in, 1 out]
  }
  n153 = Unregister For Events(event registration refnum=w10, error in=w8) -> (error out=w11:errorcluster)
  n154 = Merge Errors(w11, w14) -> (w12:errorcluster)
  n155 = call "Destroy User Event - Stop.vi"("error in (no error)"=w12, "User Event - Stop"=w3) -> ("error out"=w9:errorcluster)  [unwired: 9 in]
  n156 = disable-structure shown="RUN_TIME_ENGINE==True" {
    disable-tunnel: w9 -> [_ _]
    frame condition #0 (active) {
    }
    frame condition #1 {
      # "Call Quit LabVIEW if running as a built application."
      n157 = Quit LabVIEW() -> ()  [unwired: 1 in]
    }
  }
